vi "Auth_Token.vi"(8 "error in (no error)":errorcluster, 11 "ByteGSAPIBase in":refnum<class "ByteRESTBase.lvclass">) -> (0 "error out":errorcluster, 3 "ByteGSAPIBase out":refnum<class "ByteRESTBase.lvclass">)   [LabVIEW 2019, in "ByteREST.lvlib" / "ByteRESTBase.lvclass"]
doc: "Apre una nuova connessione HTTP e setta il content type a \"application/json\""
uses:
  ByteRESTBase.lvclass
  ByteRESTBase.lvclass/ByteRESTBase.ctl
  <vilib>/httpClient/LabVIEWHTTPClient.lvlib
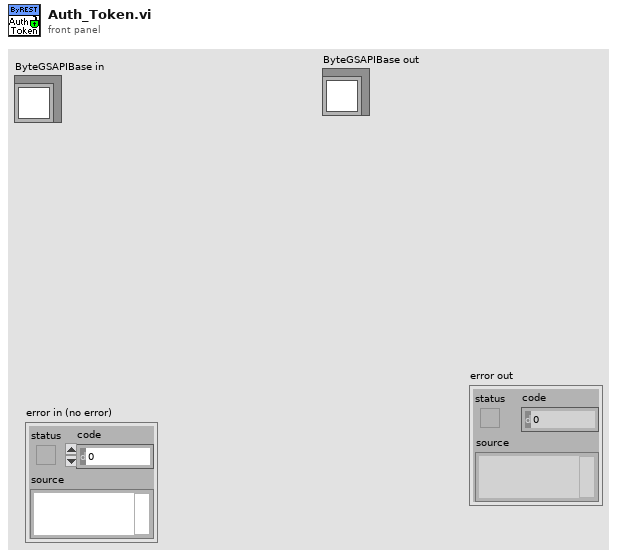
[diagram p1: front panel]
types:
  T1 = typedef "LabVIEWHTTPClient.lvlib/ClientHandle.ctl" = refnum<k1>
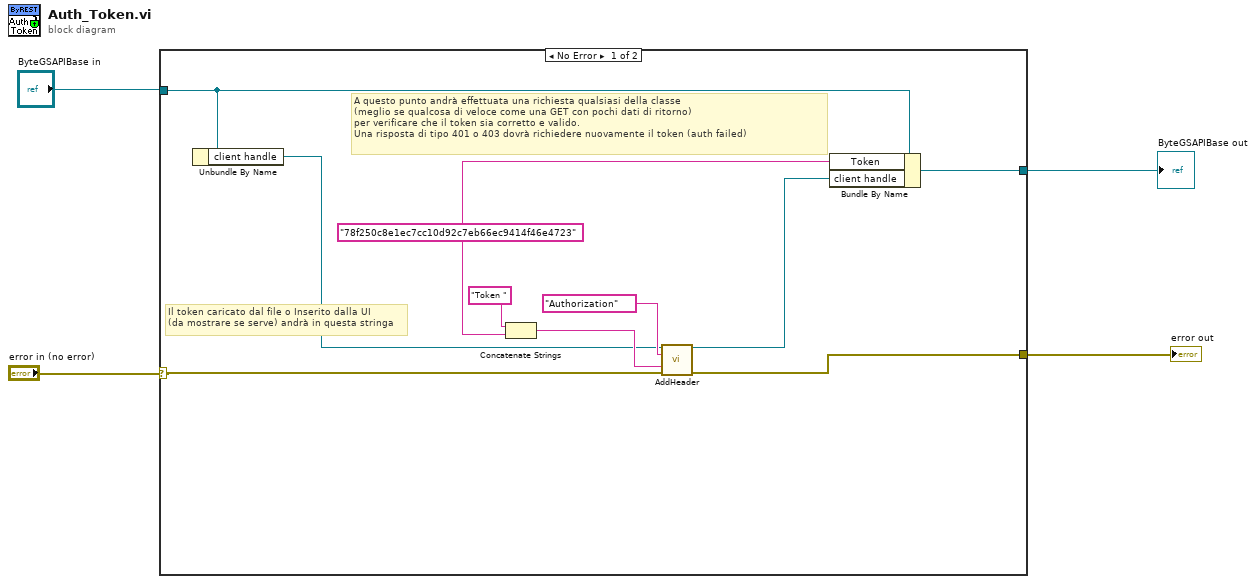
[diagram p0: block diagram]
diagram:
  n1 = case shown="No Error" "error in (no error)" {
    selector: "error in (no error)" -> [w7 w16]
    tunnel: [w9 w16] -> w3
    tunnel: [w14 w15] -> w1
    tunnel: "ByteGSAPIBase in" -> [w6 w15]
    frame No Error {
      w10 = "78f250c8e1ec7cc10d92c7eb66ec9414f46e4723"
      # "A questo punto andrà effettuata una richiesta qualsiasi della classe\n(meglio se qualcosa di veloce come una GET con pochi dati di ritorno)\nper verificare che il token sia corretto e valido.\nUna risposta di tipo 401 o 403 dovrà richiedere nuovamente il token (auth failed)"
      # "Il token caricato dal file o Inserito dalla UI\n(da mostrare se serve) andrà in questa stringa"
      n2 = Unbundle By Name(w6) -> ("client handle"=w5:T1)
      n3 = Concatenate Strings("Token " ("string"), w10) -> (w12:string)
      n4 = call <vilib>:"AddHeader.vi"("client handle"=w5, "header"="Authorization", "value"=w12, "error in (no error)"=w7) -> ("client handle out"=w8:T1, "error out"=w9:errorcluster)  [unwired: 10 in]
      n5 = Bundle By Name(cluster=w6, "Token"=w10, "client handle"=w8) -> (w14:refnum<class "ByteRESTBase.lvclass">)
    }
    frame Error {
    }
  }
  "error out" <- w3
  "ByteGSAPIBase out" <- w1
